vi "Prepare Self-address.vi"(8 "error in (no error)":errorcluster, 9 "Reply to me":refnum<class "Result Reply Msg.lvclass">, 10 "Reply to":refnum<class "Result Reply Msg.lvclass">, 11 "Measure Controller in":refnum<class "Measure Controller.lvclass">) -> (0 "error out":errorcluster, 1 "Reply to me":refnum<class "Result Reply Msg.lvclass">, 2 "Active measurements enqueuers":refnum<class "Message Enqueuer.lvclass">[](array[class]), 3 "Measure Controller out":refnum<class "Measure Controller.lvclass">)   [LabVIEW 2015, in "Measure Controller.lvclass"]
uses:
  Measure Controller.lvclass
  Measure Object Messages/Result Reply Msg/Result Reply Msg.lvclass
  <vilib>/ActorFramework/Message Enqueuer/Message Enqueuer.lvclass
  Measure Object/Measure Object.lvclass/Measure Object.ctl
  <vilib>/ActorFramework/Actor/Actor.lvclass/Actor.ctl
  <vilib>/ActorFramework/Message Enqueuer/Message Enqueuer.lvclass/Message Enqueuer.ctl
  Measure Controller.lvclass/Measure Controller.ctl
  Measure Object Messages/Self-Addressed Msg/Self-addressed Msg.lvclass/Self-addressed Msg.ctl
  Measure Object/Write Counter.vi
  Measure Object/Write Reply to.vi
  Measure Object Messages/Self-Addressed Msg/Write Return Enqueuer.vi
  <vilib>/ActorFramework/Message Enqueuer/Init from Existing Queue.vi
  <vilib>/ActorFramework/Actor/Actor.lvclass
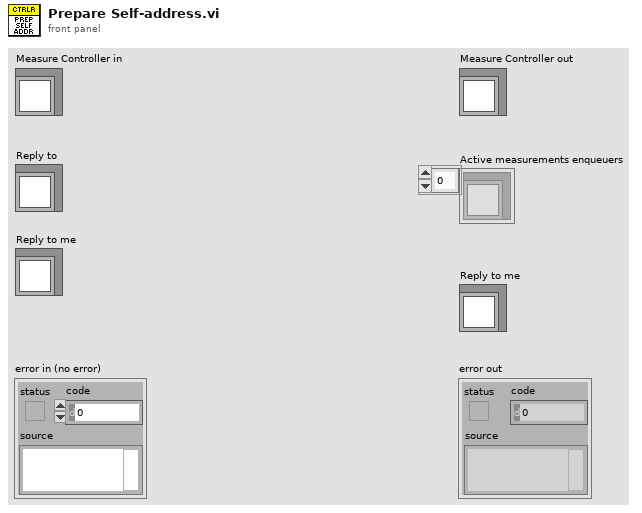
[diagram p1: front panel]
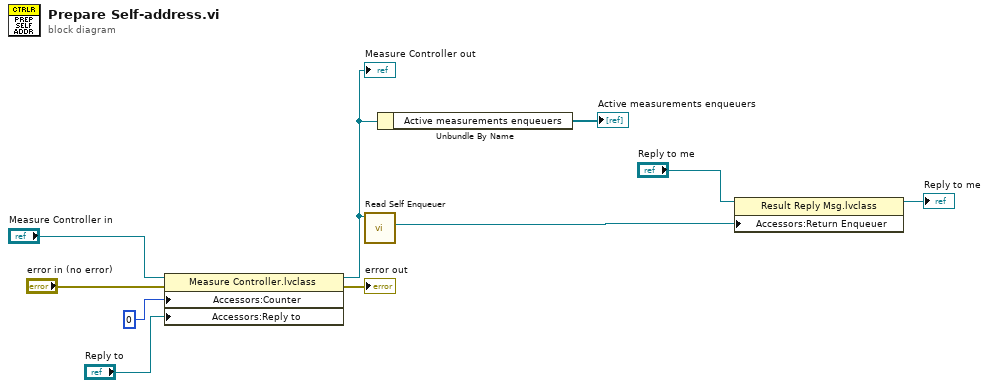
[diagram p0: block diagram]
diagram:
  n1 = property class="Measure Controller.lvclass"(reference="Measure Controller in", error in="error in (no error)", "Accessors:Counter"=0 ("Counter"), "Accessors:Reply to"="Reply to") -> (reference out=w6:refnum<class "Measure Controller.lvclass">, error out=→"error out":errorcluster)
  "Measure Controller out" <- w6
  n2 = call <vilib>:"Read Self Enqueuer.vi"("Actor"=w6) -> ("Self Enqueuer"=w4:refnum<class "Message Enqueuer.lvclass">)  [unwired: 10 in]
  n3 = Unbundle By Name(w6) -> ("Active measurements enqueuers"=→"Active measurements enqueuers":refnum<class "Message Enqueuer.lvclass">[])
  n4 = property class="Result Reply Msg.lvclass"(reference="Reply to me", "Accessors:Return Enqueuer"=w4) -> (reference out=→"Reply to me":refnum<class "Result Reply Msg.lvclass">)  [unwired: 1 in, 1 out]
